vi "Configure Export Signal.vi"(8 "error in (no error)":errorcluster, 11 "FGen Base CFG in":refnum<class "FGen Base CFG.lvclass">) -> (0 "error out":errorcluster, 3 "FGen Base CFG out":refnum<class "FGen Base CFG.lvclass">)   [LabVIEW 2023, in "FGen Base CFG.lvclass"]
uses:
  FGen Base CFG.lvclass
  FGen Base CFG.lvclass/FGen Base CFG.ctl
  <vilib>/Utility/error.llb/Error Cluster From Error Code.vi
  <vilib>/ErrorRing/Error Ring.xnode
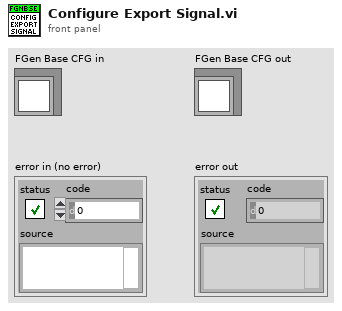
[diagram p1: front panel]
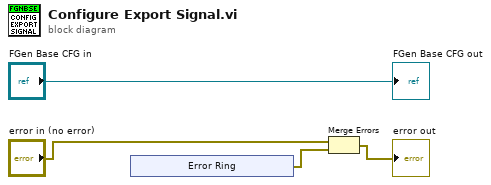
[diagram p0: block diagram]
diagram:
  n1 = xnode "Error Ring"() -> ("error out"=w3:errorcluster)
  n2 = Merge Errors("error in (no error)", w3) -> (→"error out":errorcluster)
  "FGen Base CFG out" <- "FGen Base CFG in"
